vi "addPreamble.vi"(0 "Input Symbol Stream":cdb[][](array[numeric]), 7 "Training Sequence":cdb[](array[numeric])=[0.7071067811865475+0.7071067811865475i, 0.7071067811865475+0.7071067811865475i, 0.7071067811865475+0.7071067811865475i, -0.7071067811865475-0.7071067811865475i, -0.7071067811865475-0.7071067811865475i, -0.7071067811865475-0.7071067811865475i, 0.7071067811865475+0.7071067811865475i, -0.7071067811865475-0.7071067811865475i, -0.7071067811865475-0.7071067811865475i, 0.7071067811865475+0.7071067811865475i, -0.7071067811865475-0.7071067811865475i, 0.7071067811865475+0.7071067811865475i, 0.7071067811865475+0.7071067811865475i, 0.7071067811865475+0.7071067811865475i, -0.7071067811865475-0.7071067811865475i, -0.7071067811865475-0.7071067811865475i, -0.7071067811865475-0.7071067811865475i, 0.7071067811865475+0.7071067811865475i, -0.7071067811865475-0.7071067811865475i, -0.7071067811865475-0.7071067811865475i, 0.7071067811865475+0.7071067811865475i, -0.7071067811865475-0.7071067811865475i, 0.7071067811865475+0.7071067811865475i, 0.7071067811865475+0.7071067811865475i, 0.7071067811865475+0.7071067811865475i, -0.7071067811865475-0.7071067811865475i, -0.7071067811865475-0.7071067811865475i, -0.7071067811865475-0.7071067811865475i, 0.7071067811865475+0.7071067811865475i, -0.7071067811865475-0.7071067811865475i, -0.7071067811865475-0.7071067811865475i, 0.7071067811865475+0.7071067811865475i, -0.7071067811865475-0.7071067811865475i, 0.7071067811865475+0.7071067811865475i, 0.7071067811865475+0.7071067811865475i, 0.7071067811865475+0.7071067811865475i, -0.7071067811865475-0.7071067811865475i, -0.7071067811865475-0.7071067811865475i, -0.7071067811865475-0.7071067811865475i, 0.7071067811865475+0.7071067811865475i, -0.7071067811865475-0.7071067811865475i, -0.7071067811865475-0.7071067811865475i, 0.7071067811865475+0.7071067811865475i, -0.7071067811865475-0.7071067811865475i] format="%#_3p", 9 "Training Sequence 2":cdb[](array[numeric])=[0.7071067811865475+0.7071067811865475i, 0.7071067811865475+0.7071067811865475i, 0.7071067811865475+0.7071067811865475i, -0.7071067811865475-0.7071067811865475i, -0.7071067811865475-0.7071067811865475i, -0.7071067811865475-0.7071067811865475i, 0.7071067811865475+0.7071067811865475i, -0.7071067811865475-0.7071067811865475i, -0.7071067811865475-0.7071067811865475i, 0.7071067811865475+0.7071067811865475i, -0.7071067811865475-0.7071067811865475i, 0.7071067811865475+0.7071067811865475i, 0.7071067811865475+0.7071067811865475i, 0.7071067811865475+0.7071067811865475i, -0.7071067811865475-0.7071067811865475i, -0.7071067811865475-0.7071067811865475i, -0.7071067811865475-0.7071067811865475i, 0.7071067811865475+0.7071067811865475i, -0.7071067811865475-0.7071067811865475i, -0.7071067811865475-0.7071067811865475i, 0.7071067811865475+0.7071067811865475i, -0.7071067811865475-0.7071067811865475i, 0.7071067811865475+0.7071067811865475i, 0.7071067811865475+0.7071067811865475i, 0.7071067811865475+0.7071067811865475i, -0.7071067811865475-0.7071067811865475i, -0.7071067811865475-0.7071067811865475i, -0.7071067811865475-0.7071067811865475i, 0.7071067811865475+0.7071067811865475i, -0.7071067811865475-0.7071067811865475i, -0.7071067811865475-0.7071067811865475i, 0.7071067811865475+0.7071067811865475i, -0.7071067811865475-0.7071067811865475i, 0.7071067811865475+0.7071067811865475i, 0.7071067811865475+0.7071067811865475i, 0.7071067811865475+0.7071067811865475i, -0.7071067811865475-0.7071067811865475i, -0.7071067811865475-0.7071067811865475i, -0.7071067811865475-0.7071067811865475i, 0.7071067811865475+0.7071067811865475i, -0.7071067811865475-0.7071067811865475i, -0.7071067811865475-0.7071067811865475i, 0.7071067811865475+0.7071067811865475i, -0.7071067811865475-0.7071067811865475i] format="%#_3p", 11 "error in (no error)":errorcluster) -> (4 "Output Transmit \nPackets":cdb[][](array[numeric]), 15 "error out":errorcluster)   [LabVIEW 2014]
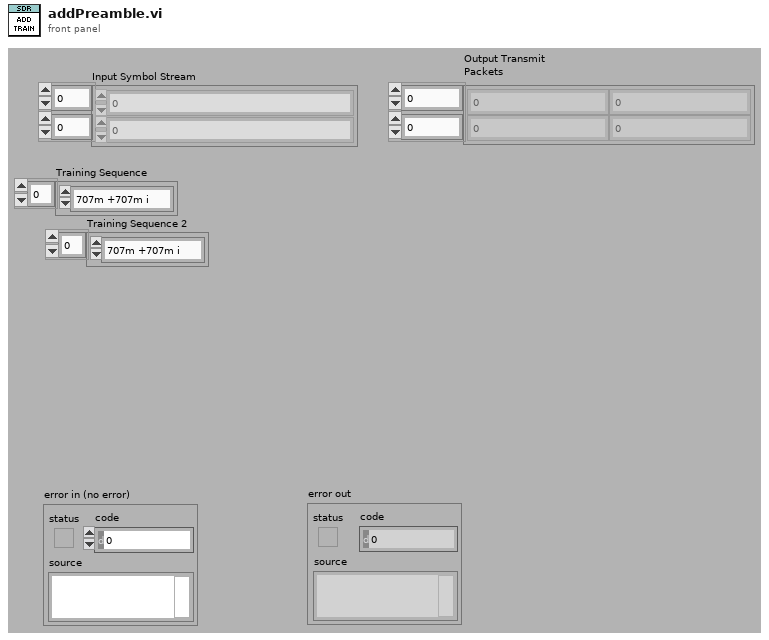
[diagram p1: front panel]
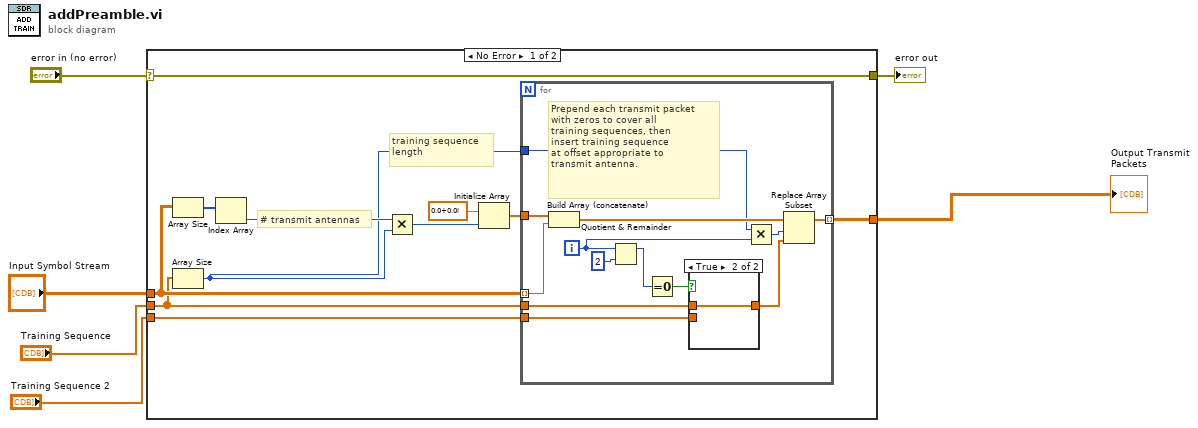
[diagram p0: block diagram]
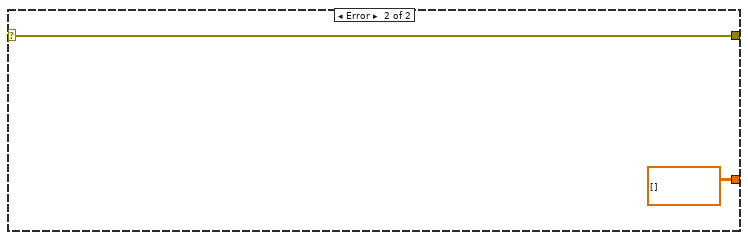
[diagram p3: hidden frame]
diagram:
  n1 = case shown="No Error" "error in (no error)" {
    selector: "error in (no error)" -> [w17 w34]
    tunnel: [w17 w34] -> w5
    tunnel: "Input Symbol Stream" -> [w15 _]
    tunnel: "Training Sequence" -> [w9 _]
    tunnel: [w7 cdb[][] []] -> w1
    tunnel: "Training Sequence 2" -> [w8 _]
    frame No Error {
      # "training sequence\nlength"
      # "# transmit antennas"
      n2 = Array Size(array=w15) -> (size(s)=w14:i32[])
      n3 = Array Size(array=w9) -> (size(s)=w10:i32)
      n4 = Index Array(array=w14) -> (element=w13:i32)  [unwired: 1 in]
      n5 = Multiply(x=w13, y=w10) -> (x*y=w12:i32)
      n6 = Initialize Array(cdb 0.0+0.0i, w12) -> (w11:cdb[])
      n7 = for {
        tunnel: w15 -> [w29] mode=indexing
        tunnel: w11 -> [w30]
        tunnel: w10 -> [w27]
        tunnel: w9 -> [w21]
        tunnel: [w25] -> w7 mode=indexing
        tunnel: w8 -> [w19]
        i -> [w24]
        # "Prepend each transmit packet\nwith zeros to cover all\ntraining sequences, then \ninsert training sequence\nat offset appropriate to \ntransmit antenna."
        n8 = Build Array (concatenate)(w30, w29) -> (w28:cdb[])
        n9 = Quotient & Remainder(x=w24, y=2) -> (x-y*floor(x/y)=w18:i32)  [unwired: 1 out]
        n10 = Equal To 0?(x=w18) -> (x = 0?=w22:bool)
        n11 = case shown="True" w22 {
          tunnel: w21 -> [_ w32]
          tunnel: [w31 w32] -> w20
          tunnel: w19 -> [w31 _]
          frame False {
          }
          frame True {
          }
        }
        n12 = Multiply(x=w27, y=w24) -> (x*y=w26:i32)
        n13 = Replace Array Subset(array=w28, new element=w20, index=w26) -> (w25:cdb[])
      }
    }
    frame Error {
    }
  }
  "error out" <- w5
  "Output Transmit \nPackets" <- w1
